vi "stepTriggerGlobalVarsWrite.vi"(0 "stepTriggerTypes":T3, 1 "selectStepTrigger":T2, 2 "step_trig_delay_10ns_ticks":u32, 3 "stepTriggerEdge":T1=enum."true-false") -> ()   [LabVIEW 2014]
uses:
  Controls/triggerTypes.ctl
  Controls/selectTrigger.ctl
  Controls/triggerEdge.ctl
  <vilib>/rvi/Emulation/niFpgaSctlEmulationGetInTimedLoop.vi
  stepTriggerGlobalVars.vi
  <vilib>/rvi/Emulation/niFpgaProcessEmulError.vi
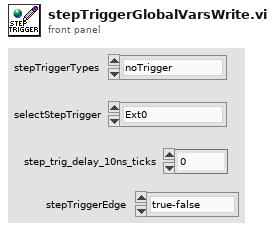
[diagram p1: front panel]
types:
  T1 = typedef "triggerEdge.ctl" = enum8{"either", "false-true", "true-false"}
  T2 = typedef "selectTrigger.ctl" = enum8{"Ext0", "Ext1", "Ext2", "Ext3", "Ext4", "Ext5", "Ext6", "Ext7", "Int0", "Int1", "Int2", "Int3", "Int4", "Int5", "Int6", "Int7"}
  T3 = typedef "triggerTypes.ctl" = enum16{"noTrigger", "singleHitDelay", "singleHit", "software", "sweep"}
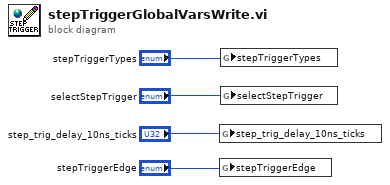
[diagram p0: block diagram]
diagram:
  n1 = global write "stepTriggerGlobalVars.vi" "step_trig_delay_10ns_ticks"("step_trig_delay_10ns_ticks") -> ()
  n2 = global write "stepTriggerGlobalVars.vi" "stepTriggerEdge"("stepTriggerEdge") -> ()
  n3 = global write "stepTriggerGlobalVars.vi" "stepTriggerTypes"("stepTriggerTypes") -> ()
  n4 = global write "stepTriggerGlobalVars.vi" "selectStepTrigger"("selectStepTrigger") -> ()
